vi "demo.vi"() -> ()   [LabVIEW 2021]
uses:
  DoublyLinkedList/DoublyLinkedList.lvclass
  DoublyNodeRef/DoublyNodeRef.lvclass
panel:
  out "error out":errorcluster
  out "data":dbl[](array[numeric])
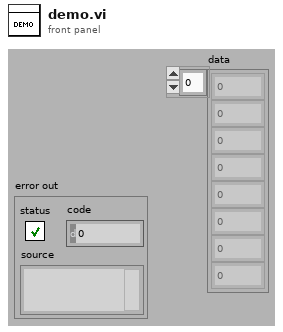
[diagram p1: front panel]
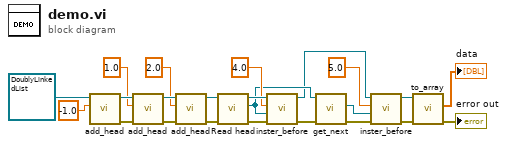
[diagram p0: block diagram]
diagram:
  n1 = call-dynamic "add_head.vi"("data"=-1.0, "DoublyLinkedList in"=refnum<class "DoublyLinkedList.lvclass"> refnum ("DoublyLinkedList.lvclass")) -> ("error out"=w18:errorcluster, "DoublyLinkedList out"=w22:refnum<class "DoublyLinkedList.lvclass">)  [unwired: 8 in]
  n2 = call-dynamic "add_head.vi"("error in (no error)"=w18, "data"=1.0, "DoublyLinkedList in"=w22) -> ("error out"=w19:errorcluster, "DoublyLinkedList out"=w21:refnum<class "DoublyLinkedList.lvclass">)  [unwired: 7 in]
  n3 = call-dynamic "add_head.vi"("error in (no error)"=w19, "data"=2.0, "DoublyLinkedList in"=w21) -> ("error out"=w5:errorcluster, "DoublyLinkedList out"=w13:refnum<class "DoublyLinkedList.lvclass">)  [unwired: 7 in]
  n4 = call-dynamic "Read head.vi"("error in (no error)"=w5, "DoublyLinkedList in"=w13) -> ("error out"=w4:errorcluster, "DoublyNodeRef.lvclass"=w10:refnum<class "DoublyNodeRef.lvclass">, "DoublyLinkedList out"=w12:refnum<class "DoublyLinkedList.lvclass">)  [unwired: 7 in]
  n5 = call-dynamic "inster_before.vi"("error in (no error)"=w4, "current node"=w10, "data"=4.0, "DoublyLinkedList in"=w12) -> ("error out"=w3:errorcluster, "DoublyLinkedList out"=w7:refnum<class "DoublyLinkedList.lvclass">)  [unwired: 6 in]
  n6 = call-dynamic "get_next.vi"("error in (no error)"=w3, "DoublyNodeRef in"=w10) -> ("error out"=w2:errorcluster, "next"=w9:refnum<class "DoublyNodeRef.lvclass">)  [unwired: 6 in, 2 out]
  n7 = call-dynamic "inster_before.vi"("error in (no error)"=w2, "current node"=w9, "data"=5.0, "DoublyLinkedList in"=w7) -> ("error out"=w1:errorcluster, "DoublyLinkedList out"=w6:refnum<class "DoublyLinkedList.lvclass">)  [unwired: 6 in]
  n8 = call-dynamic "to_array.vi"("error in (no error)"=w1, "List in"=w6) -> ("error out"=→"error out":errorcluster, "data"=→"data":dbl[])  [unwired: 7 in, 1 out]
